vi "delta phase to delta time.vi"(10 "delta phase (deg)":dbl format="%#_13g", 11 "freqency":dbl format="%#_13g") -> (3 "delta time":dbl)   [LabVIEW 2021]
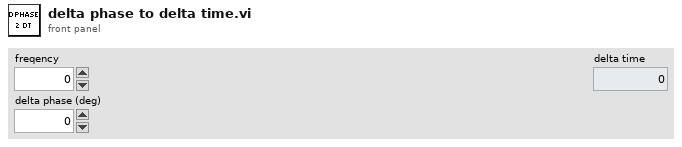
[diagram p1: front panel]
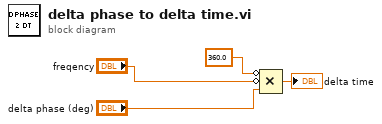
[diagram p0: block diagram]
diagram:
  n1 = Compound Arithmetic op=MULTIPLY(invert 360.0 ("value"), invert "freqency", "delta phase (deg)") -> (→"delta time":dbl)
